vi "Blue Place.vi"   [LabVIEW 2019]
uses:
  Global Var.vi
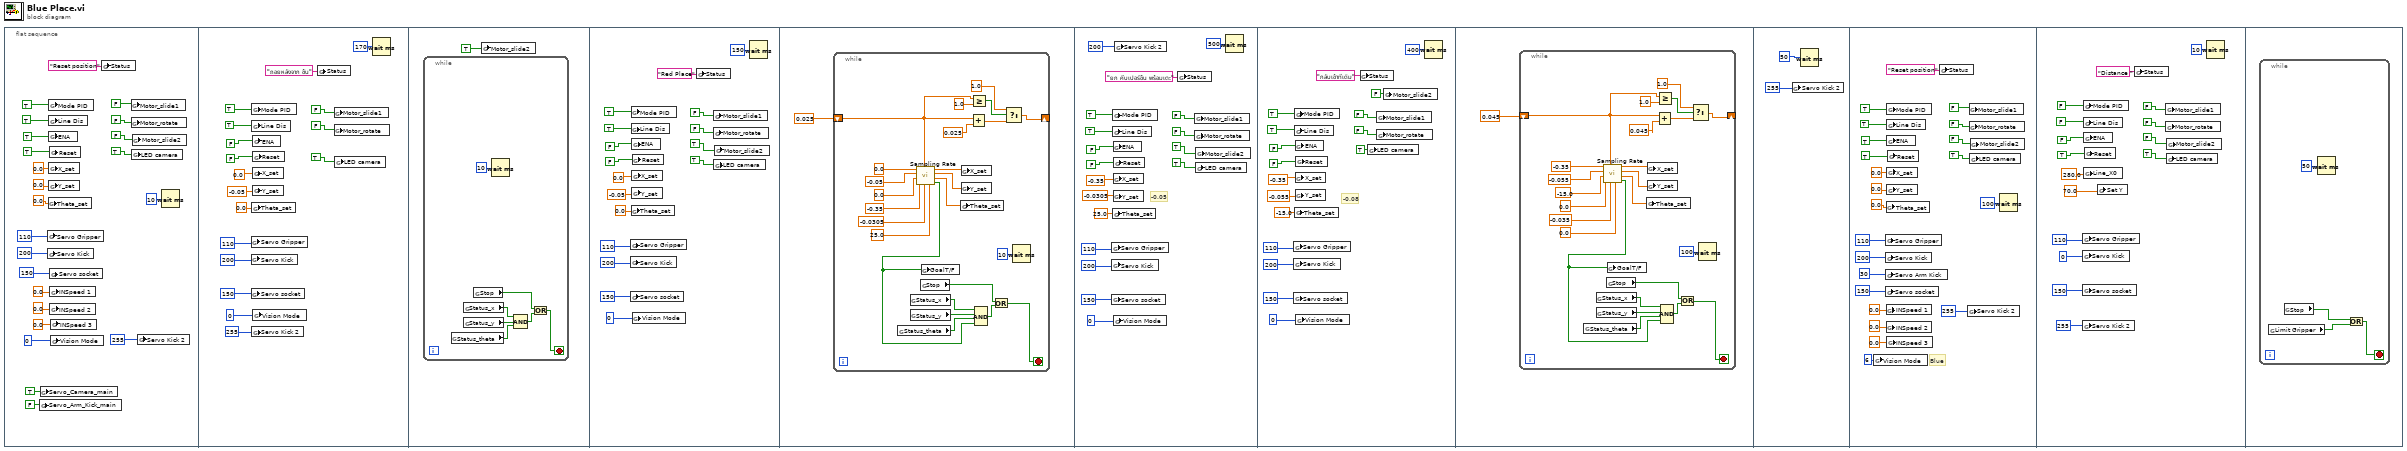
[diagram p0: block diagram]
diagram:
  n1 = flat-sequence {
    frame #0 {
      n2 = global write "Global Var.vi" "Servo_Arm_Kick_main"(FALSE ("Mode PID")) -> ()
      n3 = global write "Global Var.vi" "Servo_Camera_main"(TRUE ("Mode PID")) -> ()
      n4 = global write "Global Var.vi" "Servo Gripper"(u8 110 ("Servo Camera")) -> ()
      n5 = global write "Global Var.vi" "Servo Kick"(u8 200 ("Servo Camera")) -> ()
      n6 = global write "Global Var.vi" "Theta_set"(0.0 ("Theta_set")) -> ()
      n7 = global write "Global Var.vi" "Mode PID"(TRUE ("Mode PID")) -> ()
      n8 = global write "Global Var.vi" "Line Dis"(TRUE ("Mode PID")) -> ()
      n9 = global write "Global Var.vi" "ENA"(TRUE ("ENA")) -> ()
      n10 = global write "Global Var.vi" "X_set"(0.0 ("X_set")) -> ()
      n11 = global write "Global Var.vi" "Y_set"(0.0 ("Y_set")) -> ()
      n12 = global write "Global Var.vi" "Reset"(TRUE ("ENA")) -> ()
      n13 = global write "Global Var.vi" "Servo socket"(u8 150 ("Servo Camera")) -> ()
      n14 = global write "Global Var.vi" "INSpeed 1"(0.0 ("X_set")) -> ()
      n15 = global write "Global Var.vi" "INSpeed 2"(0.0 ("Y_set")) -> ()
      n16 = global write "Global Var.vi" "INSpeed 3"(0.0 ("Theta_set")) -> ()
      n17 = global write "Global Var.vi" "Vision Mode"(i16 0 ("Vision Mode")) -> ()
      n18 = global write "Global Var.vi" "Status"("Reset position" ("Status")) -> ()
      n19 = global write "Global Var.vi" "Motor_slide1"(FALSE ("Mode PID")) -> ()
      n20 = global write "Global Var.vi" "Motor_rotate"(FALSE ("ENA")) -> ()
      n21 = global write "Global Var.vi" "LED camera"(TRUE ("LED camera")) -> ()
      n22 = global write "Global Var.vi" "Motor_slide2"(FALSE ("ENA")) -> ()
      n23 = global write "Global Var.vi" "Servo Kick 2"(u8 255 ("Servo Camera")) -> ()
      n24 = Wait (ms)(milliseconds to wait=u32 10) -> ()  [unwired: 1 out]
    }
    frame #1 {
      n25 = global write "Global Var.vi" "Servo Gripper"(u8 110 ("Servo Camera")) -> ()
      n26 = global write "Global Var.vi" "Servo Kick"(u8 200 ("Servo Camera")) -> ()
      n27 = global write "Global Var.vi" "Servo socket"(u8 150 ("Servo Camera")) -> ()
      n28 = global write "Global Var.vi" "Mode PID"(TRUE ("Mode PID")) -> ()
      n29 = global write "Global Var.vi" "Line Dis"(TRUE ("Mode PID")) -> ()
      n30 = global write "Global Var.vi" "Theta_set"(0.0 ("Theta_set")) -> ()
      n31 = global write "Global Var.vi" "Servo Kick 2"(u8 255 ("Servo Camera")) -> ()
      n32 = global write "Global Var.vi" "ENA"(FALSE ("ENA")) -> ()
      n33 = global write "Global Var.vi" "X_set"(0.0 ("X_set")) -> ()
      n34 = global write "Global Var.vi" "Y_set"(-0.05 ("Y_set")) -> ()
      n35 = global write "Global Var.vi" "Reset"(FALSE ("ENA")) -> ()
      n36 = global write "Global Var.vi" "Vision Mode"(i16 0 ("Vision Mode")) -> ()
      n37 = global write "Global Var.vi" "Status"("ถอยหลังจาก ชั้น" ("Status")) -> ()
      n38 = global write "Global Var.vi" "Motor_slide1"(FALSE ("Mode PID")) -> ()
      n39 = global write "Global Var.vi" "Motor_rotate"(FALSE ("ENA")) -> ()
      n40 = global write "Global Var.vi" "LED camera"(TRUE ("LED camera")) -> ()
      n41 = Wait (ms)(milliseconds to wait=u32 170) -> ()  [unwired: 1 out]
    }
    frame #2 {
      n42 = while {
        stop <- w44 stop-if-true
        n43 = global read "Global Var.vi" "Status_theta"() -> (w46:bool)
        n44 = global read "Global Var.vi" "Status_x"() -> (w47:bool)
        n45 = global read "Global Var.vi" "Status_y"() -> (w48:bool)
        n46 = global read "Global Var.vi" "Stop"() -> (w42:bool)
        n47 = Wait (ms)(milliseconds to wait=u32 10) -> ()  [unwired: 1 out]
        n48 = Compound Arithmetic op=AND(w47, w48, w46) -> (w43:bool)
        n49 = Or(x=w42, y=w43) -> (x .or. y?=w44:bool)
      }
      n50 = global write "Global Var.vi" "Motor_slide2"(TRUE ("ENA")) -> ()
    }
    frame #3 {
      n51 = global write "Global Var.vi" "Servo Gripper"(u8 110 ("Servo Camera")) -> ()
      n52 = global write "Global Var.vi" "Servo Kick"(u8 200 ("Servo Camera")) -> ()
      n53 = global write "Global Var.vi" "Servo socket"(u8 150 ("Servo Camera")) -> ()
      n54 = global write "Global Var.vi" "Mode PID"(TRUE ("Mode PID")) -> ()
      n55 = global write "Global Var.vi" "Line Dis"(TRUE ("Mode PID")) -> ()
      n56 = global write "Global Var.vi" "Theta_set"(0.0 ("Theta_set")) -> ()
      n57 = global write "Global Var.vi" "ENA"(FALSE ("ENA")) -> ()
      n58 = global write "Global Var.vi" "X_set"(0.0 ("X_set")) -> ()
      n59 = global write "Global Var.vi" "Y_set"(-0.05 ("Y_set")) -> ()
      n60 = global write "Global Var.vi" "Reset"(FALSE ("ENA")) -> ()
      n61 = global write "Global Var.vi" "Vision Mode"(i16 0 ("Vision Mode")) -> ()
      n62 = global write "Global Var.vi" "Status"("Red Place" ("Status")) -> ()
      n63 = global write "Global Var.vi" "Motor_slide1"(FALSE ("Mode PID")) -> ()
      n64 = global write "Global Var.vi" "Motor_rotate"(FALSE ("ENA")) -> ()
      n65 = global write "Global Var.vi" "LED camera"(TRUE ("LED camera")) -> ()
      n66 = global write "Global Var.vi" "Motor_slide2"(TRUE ("ENA")) -> ()
      n67 = Wait (ms)(milliseconds to wait=u32 150) -> ()  [unwired: 1 out]
    }
    frame #4 {
      n68 = while {
        shift-right: [w69] -> _
        shift-left: 0.025 -> [w67]
        stop <- w86 stop-if-true
        n69 = global read "Global Var.vi" "Status_theta"() -> (w88:bool)
        n70 = global read "Global Var.vi" "Status_x"() -> (w89:bool)
        n71 = global read "Global Var.vi" "Status_y"() -> (w90:bool)
        n72 = call "Sampling Rate.vi"("input a1"=25.0, "input y1"=-0.0305, "T(0-1)"=w67, "input x1"=-0.35, "input a0"=0.0, "input y0"=-0.05, "input x0"=0.0) -> ("GoalT/F"=w74:bool, "a_output"=w81:dbl, "y_output"=w82:dbl, "x_output"=w83:dbl)  [unwired: 1 in]
        n73 = global read "Global Var.vi" "Stop"() -> (w84:bool)
        n74 = global write "Global Var.vi" "GoalT/F"(w74) -> ()
        n75 = global write "Global Var.vi" "Theta_set"(w81) -> ()
        n76 = global write "Global Var.vi" "X_set"(w83) -> ()
        n77 = global write "Global Var.vi" "Y_set"(w82) -> ()
        n78 = Add(x=w67, y=0.025) -> (x+y=w72:dbl)
        n79 = Greater Or Equal?(x=w67, y=1.0) -> (x >= y?=w71:bool)
        n80 = Compound Arithmetic op=AND(w89, w90, w88, w74) -> (w85:bool)
        n81 = Or(x=w84, y=w85) -> (x .or. y?=w86:bool)
        n82 = Select(t=1.0, s=w71, f=w72) -> (s? t:f=w69:dbl)
        n83 = Wait (ms)(milliseconds to wait=u32 10) -> ()  [unwired: 1 out]
      }
    }
    frame #5 {
      # "-0.05"
      n84 = global write "Global Var.vi" "Servo Gripper"(u8 110 ("Servo Camera")) -> ()
      n85 = global write "Global Var.vi" "Servo Kick"(u8 200 ("Servo Camera")) -> ()
      n86 = global write "Global Var.vi" "Servo socket"(u8 150 ("Servo Camera")) -> ()
      n87 = global write "Global Var.vi" "Mode PID"(TRUE ("Mode PID")) -> ()
      n88 = global write "Global Var.vi" "Line Dis"(TRUE ("Mode PID")) -> ()
      n89 = global write "Global Var.vi" "Theta_set"(25.0 ("Theta_set")) -> ()
      n90 = global write "Global Var.vi" "ENA"(FALSE ("ENA")) -> ()
      n91 = global write "Global Var.vi" "X_set"(-0.35 ("X_set")) -> ()
      n92 = global write "Global Var.vi" "Y_set"(-0.0305 ("Y_set")) -> ()
      n93 = global write "Global Var.vi" "Reset"(FALSE ("ENA")) -> ()
      n94 = global write "Global Var.vi" "Vision Mode"(i16 0 ("Vision Mode")) -> ()
      n95 = global write "Global Var.vi" "Servo Kick 2"(u8 200 ("Servo Camera")) -> ()
      n96 = global write "Global Var.vi" "Status"("ยก คีบเปอร์ขึ้น พร้อมเตะ" ("Status")) -> ()
      n97 = global write "Global Var.vi" "Motor_slide1"(FALSE ("Mode PID")) -> ()
      n98 = global write "Global Var.vi" "Motor_rotate"(FALSE ("ENA")) -> ()
      n99 = global write "Global Var.vi" "LED camera"(TRUE ("LED camera")) -> ()
      n100 = global write "Global Var.vi" "Motor_slide2"(TRUE ("ENA")) -> ()
      n101 = Wait (ms)(milliseconds to wait=u32 500) -> ()  [unwired: 1 out]
    }
    frame #6 {
      # "-0.08"
      n102 = global write "Global Var.vi" "Servo Gripper"(u8 110 ("Servo Camera")) -> ()
      n103 = global write "Global Var.vi" "Servo Kick"(u8 200 ("Servo Camera")) -> ()
      n104 = global write "Global Var.vi" "Servo socket"(u8 150 ("Servo Camera")) -> ()
      n105 = global write "Global Var.vi" "Mode PID"(TRUE ("Mode PID")) -> ()
      n106 = global write "Global Var.vi" "Line Dis"(TRUE ("Mode PID")) -> ()
      n107 = global write "Global Var.vi" "Theta_set"(-15.0 ("Theta_set")) -> ()
      n108 = global write "Global Var.vi" "ENA"(FALSE ("ENA")) -> ()
      n109 = global write "Global Var.vi" "X_set"(-0.35 ("X_set")) -> ()
      n110 = global write "Global Var.vi" "Y_set"(-0.055 ("Y_set")) -> ()
      n111 = global write "Global Var.vi" "Reset"(FALSE ("ENA")) -> ()
      n112 = global write "Global Var.vi" "Vision Mode"(i16 0 ("Vision Mode")) -> ()
      n113 = global write "Global Var.vi" "Status"("กลับเข้าที่เดิม" ("Status")) -> ()
      n114 = global write "Global Var.vi" "LED camera"(TRUE ("LED camera")) -> ()
      n115 = global write "Global Var.vi" "Motor_slide1"(FALSE ("Mode PID")) -> ()
      n116 = global write "Global Var.vi" "Motor_rotate"(FALSE ("ENA")) -> ()
      n117 = global write "Global Var.vi" "Motor_slide2"(FALSE ("ENA")) -> ()
      n118 = Wait (ms)(milliseconds to wait=u32 400) -> ()  [unwired: 1 out]
    }
    frame #7 {
      n119 = while {
        shift-right: [w130] -> _
        shift-left: 0.045 -> [w128]
        stop <- w146 stop-if-true
        n120 = global read "Global Var.vi" "Status_theta"() -> (w148:bool)
        n121 = global read "Global Var.vi" "Status_x"() -> (w149:bool)
        n122 = global read "Global Var.vi" "Status_y"() -> (w150:bool)
        n123 = call "Sampling Rate.vi"("input a1"=0.0, "input y1"=-0.035, "T(0-1)"=w128, "input x1"=0.0, "input a0"=-15.0, "input y0"=-0.055, "input x0"=-0.35) -> ("GoalT/F"=w134:bool, "a_output"=w141:dbl, "y_output"=w142:dbl, "x_output"=w143:dbl)  [unwired: 1 in]
        n124 = global read "Global Var.vi" "Stop"() -> (w144:bool)
        n125 = global write "Global Var.vi" "GoalT/F"(w134) -> ()
        n126 = global write "Global Var.vi" "Theta_set"(w141) -> ()
        n127 = global write "Global Var.vi" "X_set"(w143) -> ()
        n128 = global write "Global Var.vi" "Y_set"(w142) -> ()
        n129 = Add(x=w128, y=0.045) -> (x+y=w133:dbl)
        n130 = Greater Or Equal?(x=w128, y=1.0) -> (x >= y?=w132:bool)
        n131 = Compound Arithmetic op=AND(w149, w150, w148, w134) -> (w145:bool)
        n132 = Or(x=w144, y=w145) -> (x .or. y?=w146:bool)
        n133 = Select(t=1.0, s=w132, f=w133) -> (s? t:f=w130:dbl)
        n134 = Wait (ms)(milliseconds to wait=u32 100) -> ()  [unwired: 1 out]
      }
    }
    frame #8 {
      n135 = global write "Global Var.vi" "Servo Kick 2"(u8 255 ("Servo Camera")) -> ()
      n136 = Wait (ms)(milliseconds to wait=u32 50) -> ()  [unwired: 1 out]
    }
    frame #9 {
      # "Blue"
      n137 = global write "Global Var.vi" "Vision Mode"(i16 6 ("Vision Mode")) -> ()
      n138 = global write "Global Var.vi" "Servo Gripper"(u8 110 ("Servo Camera")) -> ()
      n139 = global write "Global Var.vi" "Servo Kick"(u8 200 ("Servo Camera")) -> ()
      n140 = global write "Global Var.vi" "Servo Arm Kick"(u8 30 ("Servo Camera")) -> ()
      n141 = global write "Global Var.vi" "Servo socket"(u8 150 ("Servo Camera")) -> ()
      n142 = global write "Global Var.vi" "Theta_set"(0.0 ("Theta_set")) -> ()
      n143 = global write "Global Var.vi" "INSpeed 1"(0.0 ("X_set")) -> ()
      n144 = global write "Global Var.vi" "INSpeed 2"(0.0 ("Y_set")) -> ()
      n145 = global write "Global Var.vi" "Mode PID"(TRUE ("Mode PID")) -> ()
      n146 = global write "Global Var.vi" "Line Dis"(TRUE ("Mode PID")) -> ()
      n147 = global write "Global Var.vi" "ENA"(TRUE ("ENA")) -> ()
      n148 = global write "Global Var.vi" "X_set"(0.0 ("X_set")) -> ()
      n149 = global write "Global Var.vi" "Y_set"(0.0 ("Y_set")) -> ()
      n150 = global write "Global Var.vi" "INSpeed 3"(0.0 ("Theta_set")) -> ()
      n151 = global write "Global Var.vi" "Reset"(TRUE ("ENA")) -> ()
      n152 = global write "Global Var.vi" "Status"("Reset position" ("Status")) -> ()
      n153 = global write "Global Var.vi" "Servo Kick 2"(u8 255 ("Servo Camera")) -> ()
      n154 = global write "Global Var.vi" "Motor_slide1"(FALSE ("Mode PID")) -> ()
      n155 = global write "Global Var.vi" "Motor_rotate"(FALSE ("ENA")) -> ()
      n156 = global write "Global Var.vi" "LED camera"(TRUE ("LED camera")) -> ()
      n157 = global write "Global Var.vi" "Motor_slide2"(FALSE ("ENA")) -> ()
      n158 = Wait (ms)(milliseconds to wait=u32 100) -> ()  [unwired: 1 out]
    }
    frame #10 {
      n159 = global write "Global Var.vi" "Servo Gripper"(u8 110 ("Servo Camera")) -> ()
      n160 = global write "Global Var.vi" "Servo Kick"(u8 0 ("Servo Camera")) -> ()
      n161 = global write "Global Var.vi" "Servo socket"(u8 150 ("Servo Camera")) -> ()
      n162 = global write "Global Var.vi" "Servo Kick 2"(u8 255 ("Servo Camera")) -> ()
      n163 = global write "Global Var.vi" "Mode PID"(FALSE ("Mode PID")) -> ()
      n164 = global write "Global Var.vi" "Line Dis"(FALSE ("Mode PID")) -> ()
      n165 = global write "Global Var.vi" "ENA"(FALSE ("ENA")) -> ()
      n166 = global write "Global Var.vi" "Line_X0"(280.0 ("Y_set")) -> ()
      n167 = global write "Global Var.vi" "Reset"(TRUE ("ENA")) -> ()
      n168 = global write "Global Var.vi" "Set Y"(70.0 ("Y_set")) -> ()
      n169 = global write "Global Var.vi" "Status"("Distance " ("Status")) -> ()
      n170 = global write "Global Var.vi" "Motor_slide1"(FALSE ("Mode PID")) -> ()
      n171 = global write "Global Var.vi" "Motor_rotate"(FALSE ("ENA")) -> ()
      n172 = global write "Global Var.vi" "LED camera"(TRUE ("LED camera")) -> ()
      n173 = global write "Global Var.vi" "Motor_slide2"(FALSE ("ENA")) -> ()
      n174 = Wait (ms)(milliseconds to wait=u32 10) -> ()  [unwired: 1 out]
    }
    frame #11 {
      n175 = while {
        stop <- w193 stop-if-true
        n176 = global read "Global Var.vi" "Limit Gripper"() -> (w191:bool)
        n177 = global read "Global Var.vi" "Stop"() -> (w192:bool)
        n178 = Wait (ms)(milliseconds to wait=u32 50) -> ()  [unwired: 1 out]
        n179 = Or(x=w192, y=w191) -> (x .or. y?=w193:bool)
      }
    }
  }
